vi "Queue Comms Dequeue.vi"(8 "error in (no error)":errorcluster, 11 "Timeout(ms)":i32=10) -> (0 "error out":errorcluster, 3 "element":T1)   [LabVIEW 2018, in "Inputs.lvlib"]
doc: "This subVI dequeues an element from the communications queue using the Queue Comms FGV"
uses:
  Inputs.lvlib
  Private Controls/Module Data.ctl
  Private Controls/Module Action.ctl
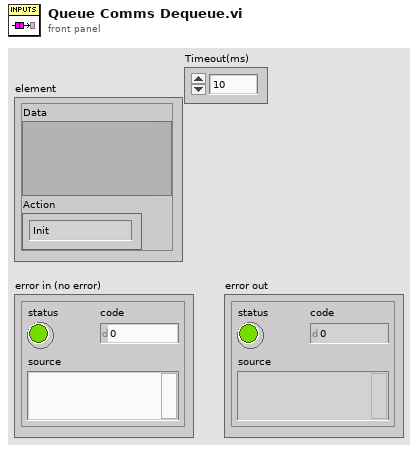
[diagram p1: front panel]
types:
  T1 = typedef "Inputs.lvlib/Module Data.ctl" = cluster{"Data":variant, "Action":T2}
  T2 = typedef "Inputs.lvlib/Module Action.ctl" = enum16{"Init", "RPMs", "Temps", "AI", "Timeout", "Error"}
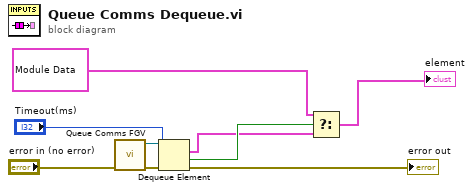
[diagram p0: block diagram]
diagram:
  n1 = call "Queue Comms FGV.vi"("error in (no error)"="error in (no error)") -> ("error out"=w8:errorcluster, "Queue out"=w7:refnum<queue>)  [unwired: 9 in]
  n2 = Dequeue Element(queue=w7, timeout in ms (-1)="Timeout(ms)", error in (no error)=w8) -> (element=w2:T1, timed out?=w4:bool, error out=→"error out":errorcluster)  [unwired: 1 out]
  n3 = Select(t=T1 {"Data"=variant, "Action"=enum."Timeout"} ("element"), s=w4, f=w2) -> (s? t:f=→"element":T1)
